vi "For Loop Scan.vi"(8 "error in (no error)":errorcluster caption="entrée d'erreur (pas d'erreur)", 10 "Pas abs(um)":dbl, 11 "UI SA en entrée":refnum<class "UI SmarAct.lvclass">) -> (0 "error out":errorcluster caption="sortie d'erreur", 2 "Reply Data out":T1, 3 "UI SA en sortie":refnum<class "UI SmarAct.lvclass">)   [LabVIEW 2024, in "UI SmarAct.lvclass"]
uses:
  UI SmarAct.lvclass
  C:/Program Files (x86)/National Instruments/LabVIEW 2024/vi.lib/addons/_Workers/Library/Classes/Worker/Worker.lvclass
  Spectro Acquisition/rwr_One Acquisition Reply.ctl
  UI SmarAct.lvclass/UI SmarAct.ctl
  79666e21-d5ce-43ca-9807-b48badf20504.vi
  Spectro Acquisition/Spectro Acquisition.lvclass
  C:/Program Files (x86)/National Instruments/LabVIEW 2024/vi.lib/addons/_Workers/Library/Classes/Workers Object/Workers Object.lvclass
  C:/Users/flepetit/Desktop/FROG-SHG-LV2024/Workers/UI SmarAct/UI SmarAct.lvclass
panel:
  out "Spectre-BKG":dbl[](array[numeric])
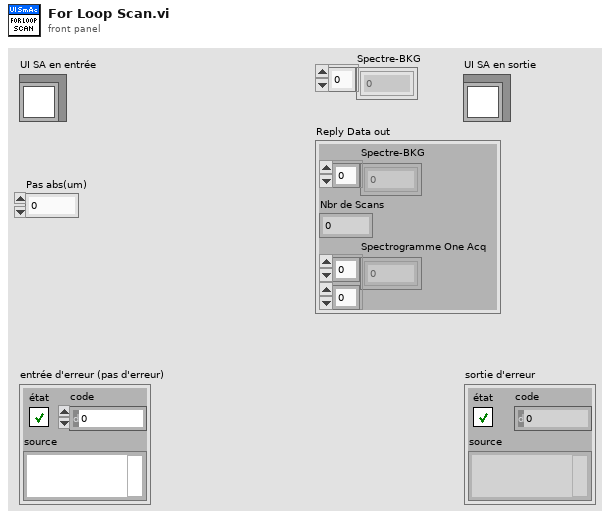
[diagram p1: front panel]
types:
  T1 = typedef "Spectro Acquisition.lvclass/rwr_One Acquisition Reply.ctl" = cluster{"Spectre-BKG":dbl[], "Nbr de Scans":i32, "Spectrogramme One Acq":dbl[][]}
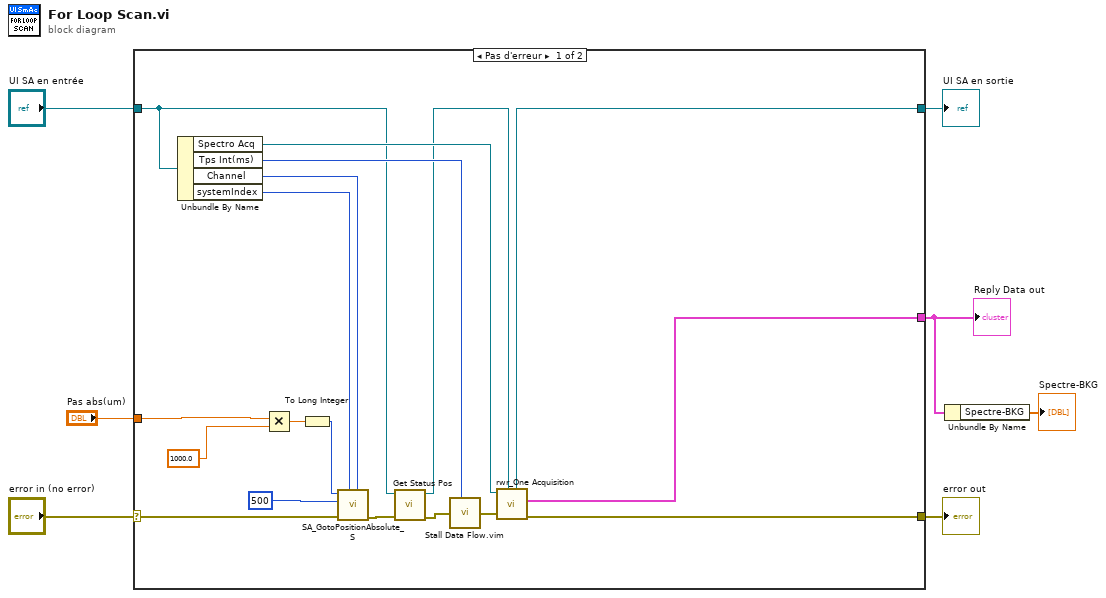
[diagram p0: block diagram]
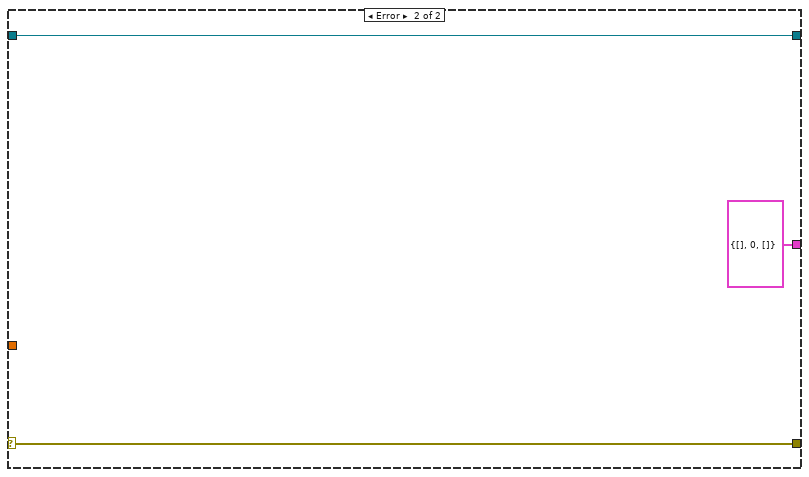
[diagram p2: hidden frame]
diagram:
  n1 = case shown="Pas d'erreur" "error in (no error)" {
    selector: "error in (no error)" -> [w22 w28]
    tunnel: [w23 w28] -> w6
    tunnel: [w12 w27] -> w4
    tunnel: "UI SA en entrée" -> [w14 w27]
    tunnel: "Pas abs(um)" -> [w10 _]
    tunnel: [w11 T1 {"Spectre-BKG"=[], "Nbr de Scans"=0, "Spectrogramme One Acq"=[]} ("Reply Data out")] -> w2
    frame No Error {
      n2 = Unbundle By Name(w14) -> ("Spectro Acq"=w15:refnum<class "Spectro Acquisition.lvclass">, "Tps Int(ms)"=w16:u32, "Channel"=w17:u32, "systemIndex"=w20:u32)
      n3 = Multiply(x=w10, y=1000.0 ("holdTime")) -> (x*y=w18:dbl)
      n4 = To Long Integer(number=w18) -> (32bit integer=w8:i32)
      n5 = call <vilib>:"SA_GotoPositionAbsolute_S.vi"("channelIndex"=w17, "systemIndex"=w20, "error in (no error)"=w22, "holdTime"=u32 500, "position"=w8) -> ("error out"=w21:errorcluster)  [unwired: 6 in]
      n6 = call "Get Status Pos.vi"("error in (no error)"=w21, "UI SA en entrée"=w14) -> ("error out"=w25:errorcluster, "UI SA en sortie"=w13:refnum<class "UI SmarAct.lvclass">)  [unwired: 8 in]
      n7 = call "Stall Data Flow.vim"("value in"=w25, "milliseconds to wait"=w16) -> ("value out"=w24:errorcluster)  [unwired: 1 out]
      n8 = call "rwr_One Acquisition.vi"("Caller in"=w13, "error in"=w24, "Spectro Acquisition in"=w15) -> ("error out"=w23:errorcluster, "Reply Data out"=w11:T1, "dup Caller out"=w12:refnum<class "UI SmarAct.lvclass">)  [unwired: 5 in, 1 out]
    }
    frame Error {
    }
  }
  "error out" <- w6
  "UI SA en sortie" <- w4
  "Reply Data out" <- w2
  n9 = Unbundle By Name(w2) -> ("Spectre-BKG"=→"Spectre-BKG":dbl[])
